vi "Get Data From TCF.vi"(0 "Session Handle in":T1, 7 "Test Conditions File":path, 11 "error in (no error)":errorcluster) -> (4 "Session Handle out":T1, 15 "error out":errorcluster)   [LabVIEW 2018, in "niRFSTS Sequence Flow.lvclass"]
uses:
  niRFSTS Sequence Flow.lvclass
  Typedefs/Session Handle.ctl
  niRFSTS Sequence Flow.lvclass/niRFSTS Sequence Flow.ctl
  Plugins/File Parsing Interface.lvlibp/File Parsing Interface.lvclass
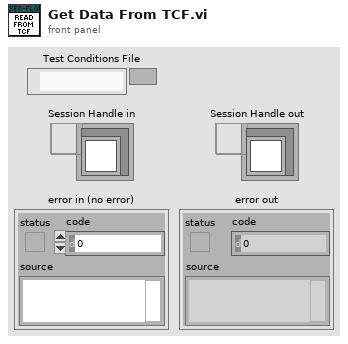
[diagram p1: front panel]
types:
  T1 = typedef "niRFSTS Sequence Flow.lvclass/Session Handle.ctl" = refnum<data-value>
  T2 = typedef "File Parsing Interface.lvlibp/File Parsing Interface.lvclass/Parsed Measurement.ctl" = cluster{"Test Mode":string, "Measurement Data Out":refnum<class "Measurement Data.lvclass">}
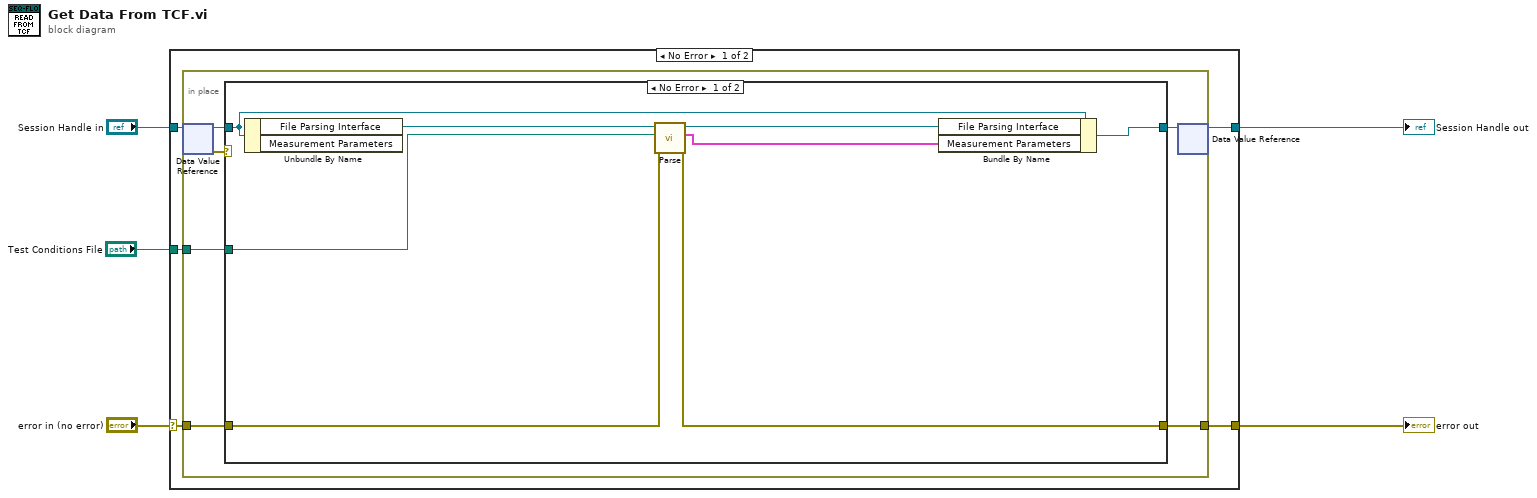
[diagram p0: block diagram]
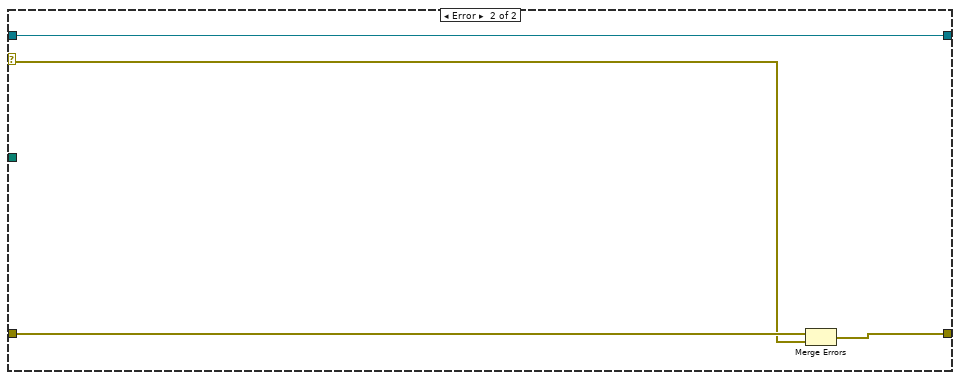
[diagram p2: hidden frame]
diagram:
  n1 = case shown="No Error" "error in (no error)" {
    selector: "error in (no error)" -> [w8 w29]
    tunnel: "Session Handle in" -> [w10 w30]
    tunnel: [w9 w30] -> w4
    tunnel: [w7 w29] -> w3
    tunnel: "Test Conditions File" -> [w6 _]
    frame No Error {
      n2 = in-place {
        in-place-border: w8 -> [w12]
        in-place-border: [w15] -> w7
        in-place-border: w6 -> [w11]
        n3 = in-place-dvr #1(w10) -> (w16:refnum<class "niRFSTS Sequence Flow.lvclass">, w13:errorcluster)
        n4 = case shown="No Error" w13 {
          selector: w13 -> [_ w27]
          tunnel: w16 -> [w24 w25]
          tunnel: [w20 w26] -> w15
          tunnel: [w23 w25] -> w14
          tunnel: w12 -> [w22 w28]
          tunnel: w11 -> [w21 _]
          frame No Error {
            n5 = Unbundle By Name(w24) -> ("File Parsing Interface"=w19:refnum<class "File Parsing Interface.lvclass">)  [unwired: 1 out]
            n6 = call-dynamic "Parse.vi"("error in (no error)"=w22, "File to Parse"=w21, "File Parsing Interface in"=w19) -> ("error out"=w20:errorcluster, "Measurements Out"=w17:T2[], "File Parsing Interface out"=w18:refnum<class "File Parsing Interface.lvclass">)  [unwired: 6 in]
            n7 = Bundle By Name(cluster=w24, "File Parsing Interface"=w18, "Measurement Parameters"=w17) -> (w23:refnum<class "niRFSTS Sequence Flow.lvclass">)
          }
          frame Error {
            n8 = Merge Errors(w28, w27) -> (w26:errorcluster)
          }
        }
        n9 = in-place-dvr #1(w14) -> (w9:T1)  [unwired: 1 out]
      }
    }
    frame Error {
    }
  }
  "Session Handle out" <- w4
  "error out" <- w3
